vi "cRIO_4DoF_Force_conversion_v2.vi"(6 "Manual force":bool, 10 "F_measured":dbl[](array[numeric]), 11 "Manual forces in":dbl[](array[numeric])) -> (2 "Force control":dbl[](array[numeric]), 3 "F_mouse":dbl[](array[numeric]))   [LabVIEW 2019]
uses:
  <vilib>/imath/engines/lvmath2/RunTimeEngine/Managers/WorkSpace/UID Generator.vi
  <vilib>/imath/engines/lvmath2/RunTimeEngine/BuiltInFunctions/size/NIMS_[I32,I32]=size(GRow).vi
  <instcachedir>/0/NIMS_[I32,I32]=size(GRow)_CFE2C4BDC5BC45CD88F2F6A295A2273D.lvgen/NIMS_[I32,I32]=size(GRow)_CFE2C4BDC5BC45CD88F2F6A295A2273D_001.vi
  <vilib>/imath/engines/lvmath2/RunTimeEngine/RunTimeType/NIMS_RunTimeType_From StrictType (excl LVString).vi
  <instcachedir>/0/NIMS_RunTimeType_From StrictType (excl LVString)_D8AFBA86A94845AAA577C895450664BD.lvgen/NIMS_RunTimeType_From StrictType (excl LVString)_D8AFBA86A94845AAA577C895450664BD_000.vi
  <vilib>/imath/engines/lvmath2/RunTimeEngine/LocalVariableDefStatement/MC_LocalVariableDefStatement_Display.vi
  <vilib>/imath/engines/lvmath2/RunTimeEngine/IndexRead/NIMS M(R2,S).vi
  <instcachedir>/0/NIMS M(R2,S)_56813DCFDD5A484292D2195AF15D2BF5.lvgen/NIMS M(R2,S)_56813DCFDD5A484292D2195AF15D2BF5_000.vi
  <vilib>/imathl/engines/lvmath/Functions/Error Handling/Create Error.vi
  <vilib>/imath/engines/lvmath2/RunTimeEngine/ArithmeticOperatorToken/NIMS_ArithmeticOperator_multmx(M,CV).vi
  <instcachedir>/0/NIMS_ArithmeticOperator_multmx(M,CV)_1D61EED49E1847F3B05DBB8EDD2FBF8F.lvgen/NIMS_ArithmeticOperator_multmx(M,CV)_1D61EED49E1847F3B05DBB8EDD2FBF8F_000.vi
  <vilib>/imath/engines/lvmath2/RunTimeEngine/IndexRead/NIMS M(S,S).vi
  <instcachedir>/0/NIMS M(S,S)_AC51E74150A542F7991B9634C66F3096.lvgen/NIMS M(S,S)_AC51E74150A542F7991B9634C66F3096_000.vi
  <vilib>/imath/engines/lvmath2/RunTimeEngine/ErrorHandling/NIMS_Create Error From Enums.vi
  <vilib>/imath/engines/lvmath2/RunTimeEngine/MatrixToken/NIMS_MatrixToken_M_SorCV.vi
  <instcachedir>/0/NIMS_MatrixToken_M_SorCV_4BD6AEBF6814499AA2FF53EAE067248B.lvgen/NIMS_MatrixToken_M_SorCV_4BD6AEBF6814499AA2FF53EAE067248B_000.vi
  <vilib>/imath/engines/lvmath2/RunTimeEngine/Managers/SymbolTable/Clear UID.vi
  <vilib>/imath/engines/lvmath2/RunTimeEngine/NodeEndStatement/NIMS_NodeEndStatement_Output.vi
  <instcachedir>/0/NIMS_NodeEndStatement_Output_53EC0D466D134D7ABD903AC30B43404B.lvgen/NIMS_NodeEndStatement_Output_53EC0D466D134D7ABD903AC30B43404B_005.vi
  <vilib>/imath/engines/lvmath2/RunTimeEngine/ErrorHandling/NIMS_Finalize Error.vi
  <vilib>/imath/engines/lvmath2/RunTimeEngine/Managers/SymbolTable/NIMS_WorkSpace.lvlib
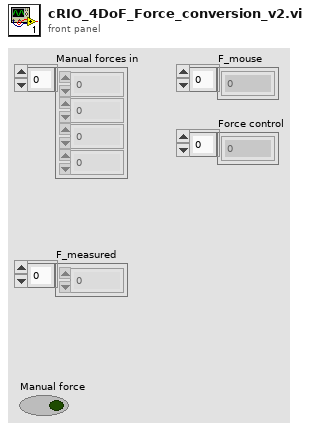
[diagram p1: front panel]
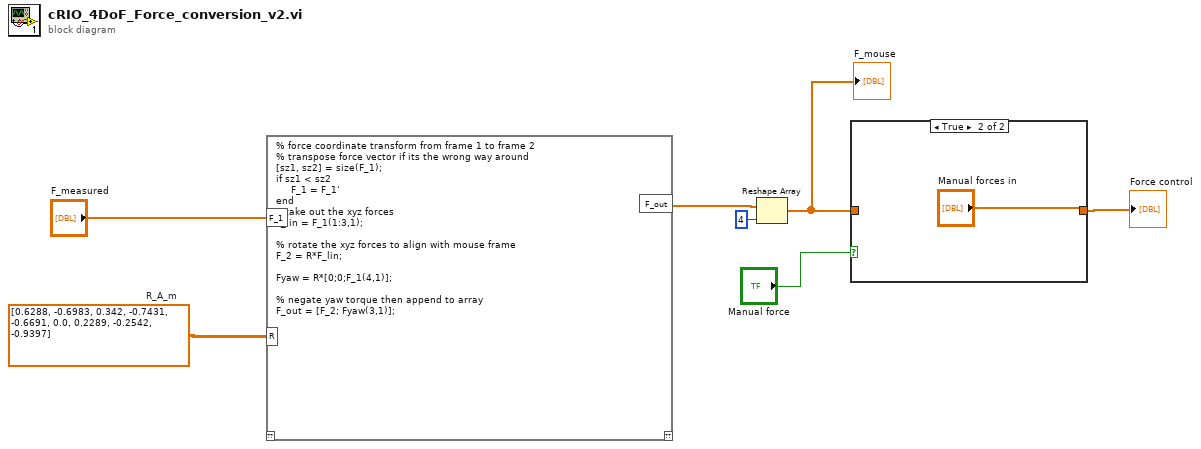
[diagram p0: block diagram]
diagram:
  w3 = dbl[][] [[0.6288, -0.6983, 0.342], [-0.7431, -0.6691, 0.0], [0.2289, -0.2542, -0.9397]]  # R_A_m
  n1 = mathscript code="% force coordinate transform from frame 1 to frame 2 \n% transpose force vector if its the wrong way around\n[sz1, sz2] = size(F_1);\nif sz1 < sz2\n     F_1 = F_1'\nend\n%take out the xyz forces\nF_lin = F_1(1:3,1);\n\n% rotate the xyz forces to align with mouse frame\nF_2 = R*F_lin;\n\nFyaw = R*[0;0;F_1(4,1)];\n\n% negate yaw torque then append to array\nF_out = [F_2; Fyaw(3,1)];"("F_1"="F_measured", "R"=w3) -> ("F_out"=w1:dbl[])  [unwired: 1 in, 1 out]
  n2 = Reshape Array(w1, 4 ("dimension size")) -> (w6:dbl[])
  "F_mouse" <- w6
  n3 = case shown="True" "Manual force" {
    tunnel: [w8 "Manual forces in"] -> w4
    tunnel: w6 -> [w8 _]
    frame False {
    }
    frame True {
    }
  }
  "Force control" <- w4
